vi "FTW-Actor-CloneName.vi"() -> (0 "Clone Name":string)   [LabVIEW 2014]
panel:
  # "Inputs"
  # "Outputs"
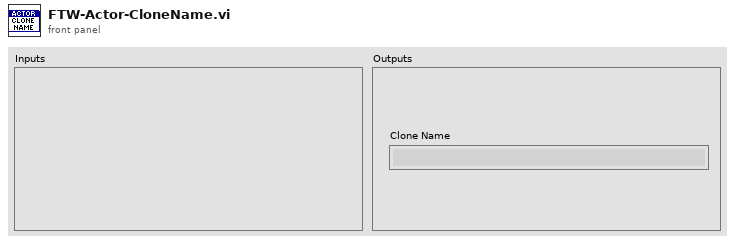
[diagram p1: front panel]
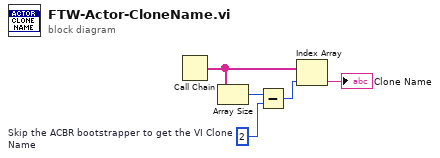
[diagram p0: block diagram]
diagram:
  w1 = 2  # Skip the ACBR bootstrapper to get the VI Clone Name
  n1 = Call Chain() -> (call chain=w3:string[])
  n2 = Array Size(array=w3) -> (size(s)=w5:i32)
  n3 = Subtract(x=w5, y=w1) -> (x-y=w4:i32)
  n4 = Index Array(array=w3, index=w4) -> (element=→"Clone Name":string)
